vi "SetRptFreq.vi"(8 "错误输入（无错误）":errorcluster, 10 "采样重复频率":sgl) -> (0 "错误输出":errorcluster)   [LabVIEW 2018]
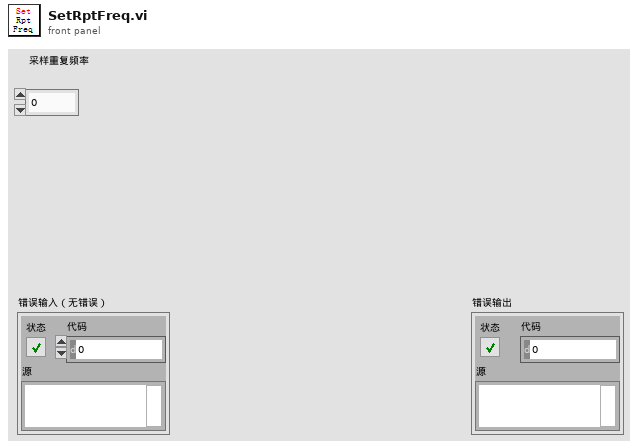
[diagram p1: front panel]
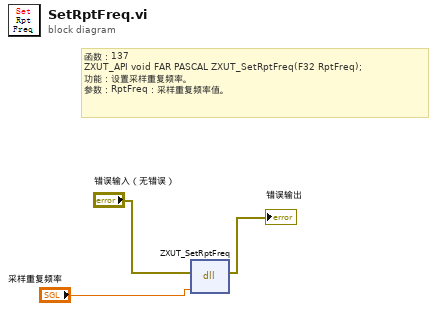
[diagram p0: block diagram]
diagram:
  # "函数：137\nZXUT_API void\tFAR PASCAL ZXUT_SetRptFreq(F32 RptFreq);\n功能：设置采样重复频率。\n参数：RptFreq：采样重复频率值。"
  n1 = dll-call lib="PTH2Rabs E软件项目超声超声子VI函数VI\tTCG处理ZXUTConfigMgr.dll" fn="ZXUT_SetRptFreq"(error in="错误输入（无错误）", "RptFreq"="采样重复频率") -> (error out=→"错误输出":errorcluster)  [unwired: 4 in, 1 out]
